vi "runtime path validation.vi"(8 "error in":errorcluster, 11 "bin datalogger configuration in":refnum<class "Binary datalogger configuration.lvclass">) -> (0 "error out":errorcluster, 3 "bin datalogger configuration out":refnum<class "Binary datalogger configuration.lvclass">)   [LabVIEW 2013, in "Binary datalogger configuration.lvclass"]
uses:
  Binary datalogger configuration.lvclass
  Binary datalogger configuration.lvclass/Binary datalogger configuration.ctl
  Write Path.vi
  Read backup directory.vi
  Write backup directory.vi
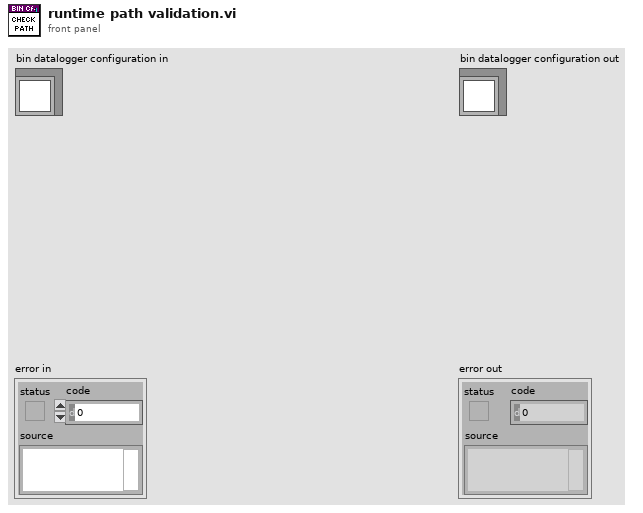
[diagram p1: front panel]
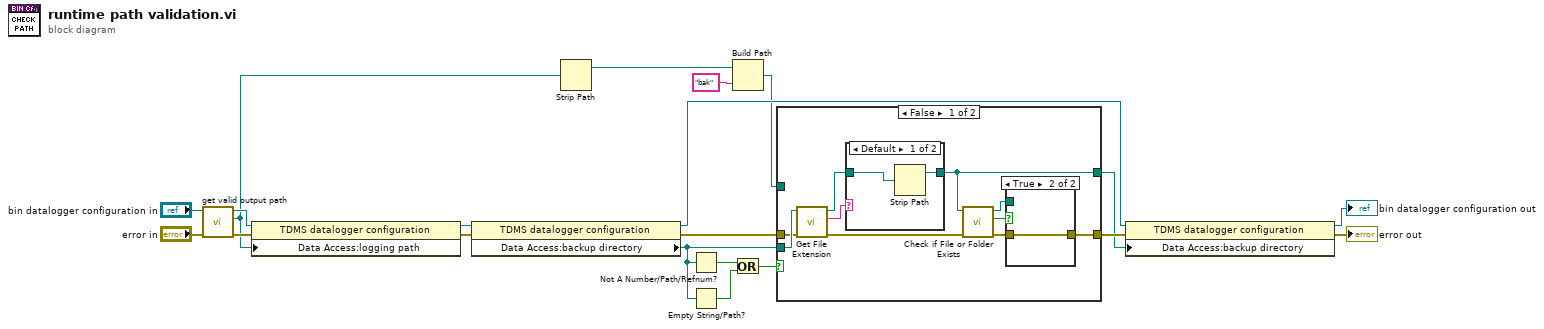
[diagram p0: block diagram]
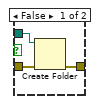
[diagram p2: hidden frame]
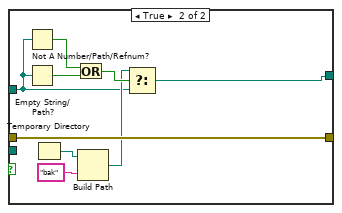
[diagram p4: hidden frame]
diagram:
  n1 = call "get valid output path.vi"("error in (no error)"="error in", "bin datalogger configuration in"="bin datalogger configuration in") -> ("error out"=w16:errorcluster, "Path"=w3:path, "bin datalogger configuration out"=w15:refnum<class "Binary datalogger configuration.lvclass">)  [unwired: 7 in]
  n2 = property class="TDMS datalogger configuration"(reference=w15, error in=w16, "Data Access:logging path"=w3) -> (reference out=w18:refnum<class "Binary datalogger configuration.lvclass">, error out=w17:errorcluster)
  n3 = property class="TDMS datalogger configuration"(reference=w18, error in=w17) -> (reference out=w6:refnum<class "Binary datalogger configuration.lvclass">, error out=w10:errorcluster, "Data Access:backup directory"=w11:path)
  n4 = Strip Path(path=w3) -> (stripped path=w4:path)  [unwired: 1 out]
  n5 = Not A Number/Path/Refnum?(number/path/refnum=w11) -> (NaN/Path/Refnum?=w13:bool)
  n6 = Empty String/Path?(string/path=w11) -> (empty?=w14:bool)
  n7 = Build Path(base path=w4, name or relative path="bak") -> (appended path=w1:path)
  n8 = Or(x=w13, y=w14) -> (x .or. y?=w12:bool)
  n9 = case shown="False" w12 {
    tunnel: [w21 w40] -> w8
    tunnel: [w26 w45] -> w9
    tunnel: w11 -> [w23 _]
    tunnel: w10 -> [w22 w45]
    tunnel: w1 -> [_ w39]
    frame False {
      n10 = call <vilib>:"Get File Extension.vi"("error in (no error)"=w22, "file"=w23) -> ("error out"=w28:errorcluster, "lowercase file extension"=w29:string, "dup file"=w30:path)  [unwired: 6 in, 1 out]
      n11 = case shown="Default" w29 {
        tunnel: w30 -> [w36 w37]
        tunnel: [w35 w37] -> w21
        frame Default {
          n12 = Strip Path(path=w36) -> (stripped path=w35:path)  [unwired: 1 out]
        }
        frame "" {
        }
      }
      n13 = call <vilib>:"Check if File or Folder Exists.vi"("error in (no error)"=w28, "path"=w21) -> ("error out"=w25:errorcluster, "file or folder exists?"=w27:bool, "dup path"=w24:path)  [unwired: 7 in]
      n14 = case shown="True" w27 {
        tunnel: [w31 w34] -> w26
        tunnel: w25 -> [w32 w34]
        tunnel: w24 -> [w33 _]
        frame False {
          n15 = Create Folder(path (use dialog)=w33, error in=w32) -> (error out=w31:errorcluster)  [unwired: 1 in, 2 out]
        }
        frame True {
        }
      }
    }
    frame True {
      n16 = Not A Number/Path/Refnum?(number/path/refnum=w39) -> (NaN/Path/Refnum?=w44:bool)
      n17 = Empty String/Path?(string/path=w39) -> (empty?=w43:bool)
      n18 = Temporary Directory() -> (w46:path)
      n19 = Or(x=w44, y=w43) -> (x .or. y?=w42:bool)
      n20 = Build Path(base path=w46, name or relative path="bak") -> (appended path=w41:path)
      n21 = Select(t=w41, s=w42, f=w39) -> (s? t:f=w40:path)
    }
  }
  n22 = property class="TDMS datalogger configuration"(reference=w6, error in=w9, "Data Access:backup directory"=w8) -> (reference out=→"bin datalogger configuration out":refnum<class "Binary datalogger configuration.lvclass">, error out=→"error out":errorcluster)
